vi "RingItemSet.vi"(7 "Target":refnum<vi>, 9 "Value":i32, 10 "Base":refnum<vi>) -> ()   [LabVIEW 2017]
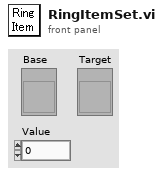
[diagram p1: front panel]
types:
  T1 = typedef "LVStringsAndValuesArrayTypeDef.ctl" = cluster{"String":string, "Value":ext}[]
  T2 = enum8{"Enabled", "Disabled", "Disabled and Grayed Out"}
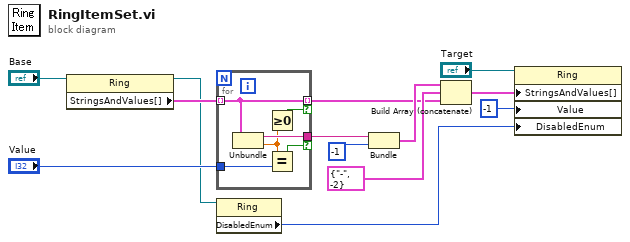
[diagram p0: block diagram]
diagram:
  n1 = property class="Ring"(reference="Base") -> (reference out=w2:refnum<vi>, "StringsAndValues[]"=w4:T1)  [unwired: 1 in, 1 out]
  n2 = for {
    tunnel: "Value" -> [w19]
    tunnel: [w18] -> w11 if=w14
    tunnel: w4 -> [w17] mode=indexing
    tunnel: [w17] -> w3 mode=indexing if=w15
    n3 = Unbundle(w17) -> ("String"=w18:string, "Value"=w16:ext)
    n4 = Greater Or Equal To 0?(x=w16) -> (x >= 0?=w15:bool)
    n5 = Equal?(x=w16, y=w19) -> (x = y?=w14:bool)
  }
  n6 = property class="Ring"(reference=w2) -> ("DisabledEnum"=w1:T2)  [unwired: 1 in, 2 out]
  n7 = Bundle("String"=w11, -1) -> (w9:cluster{"String":string, i32})  [unwired: 1 in]
  n8 = Build Array (concatenate)(w9, cluster{"String":string, i32} {"String"="-", -2} ("output cluster"), w3) -> (w7:cluster{"String":string, "Value":ext}[])
  n9 = property class="Ring"(reference="Target", "StringsAndValues[]"=w7, "Value"=-1, "DisabledEnum"=w1) -> ()  [unwired: 1 in, 2 out]
